vi "Configure Channel (Auto Threshold Voltage).vi"(6 "Percent (50 Percent )":dbl=50.0, 7 "Event Type (1: Start)":i32(ring)=1 items=["Start"=1, "Stop"=2], 8 "error in (no error)":errorcluster, 9 "Enable Auto-leveling (1: ON)":i32(ring)=1 items=["OFF", "ON", "ONCE"], 10 "Channel (1: Channel 1)":i32(ring)=1 items=["Channel 1"=1, "Channel 2"=2], 11 "VISA resource name":refnum<visa-resource-name>) -> (0 "error out":errorcluster, 3 "VISA resource name out":refnum<visa-resource-name>)   [LabVIEW 2024, in "Agilent 532XX Series.lvlib"]
doc: "Configures the threshold voltage characteristics of input channel with the auto-leveling enabled."
uses:
  Agilent 532XX Series.lvlib
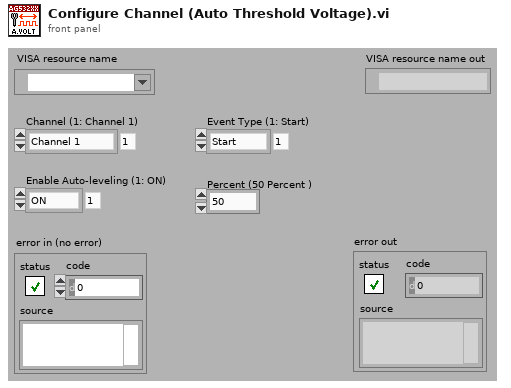
[diagram p1: front panel]
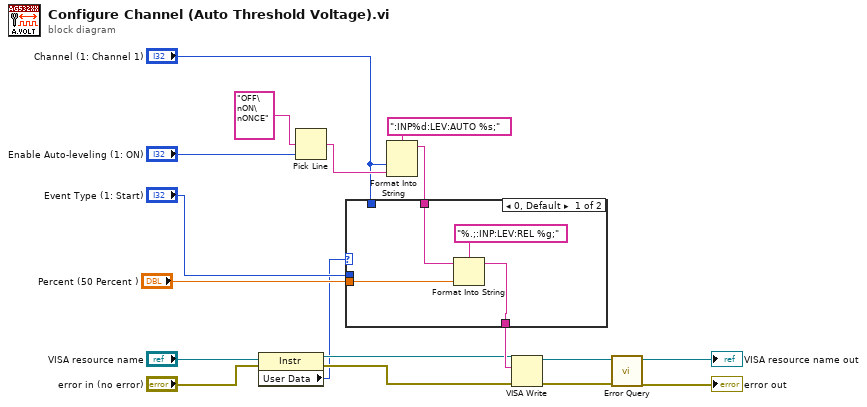
[diagram p0: block diagram]
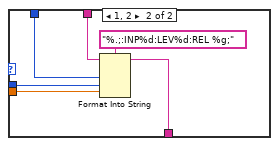
[diagram p2: hidden frame]
diagram:
  n1 = property class="Instr"(reference="VISA resource name", error in="error in (no error)") -> (reference out=w5:refnum<visa-resource-name>, error out=w3:errorcluster, "User Data"=w2:u32)
  n2 = Pick Line(multi-line string="OFF\nON\nONCE", line index="Enable Auto-leveling (1: ON)") -> (output string=w15:string)  [unwired: 1 out]
  n3 = Format Into String(format string=":INP%d:LEV:AUTO %s;", "Channel (1: Channel 1)", w15) -> (resulting string=w14:string)  [unwired: 2 in, 1 out]
  n4 = case shown="0, Default" w2 {
    tunnel: w14 -> [w20 w28]
    tunnel: "Event Type (1: Start)" -> [_ w26]
    tunnel: [w19 w25] -> w12
    tunnel: "Percent (50 Percent )" -> [w21 w24]
    tunnel: "Channel (1: Channel 1)" -> [_ w23]
    frame 0, Default {
      n5 = Format Into String(format string="%.;:INP:LEV:REL %g;", initial string=w20, w21) -> (resulting string=w19:string)  [unwired: 1 in, 1 out]
    }
    frame 1, 2 {
      n6 = Format Into String(format string="%.;:INP%d:LEV%d:REL %g;", initial string=w28, w23, w26, w24) -> (resulting string=w25:string)  [unwired: 1 in, 1 out]
    }
  }
  n7 = VISA Write(VISA resource name=w5, write buffer=w12, error in (no error)=w3) -> (VISA resource name out=w11:refnum<visa-resource-name>, error out=w10:errorcluster)  [unwired: 1 out]
  n8 = call "Error Query.vi"("error in (no error)"=w10, "VISA resource name"=w11) -> ("error out"=→"error out":errorcluster, "VISA resource name out"=→"VISA resource name out":refnum<visa-resource-name>)  [unwired: 8 out]
